vi "Load JSON Double.vi"(7 "Element":string, 8 "error in (no error)":errorcluster, 10 "Section":string, 11 "JSON string":string) -> (0 "error out":errorcluster, 3 "value":dbl)   [LabVIEW 2026, in "Settings Service.lvclass"]
uses:
  Settings Service.lvclass
  Settings Service.lvclass/Settings Service.ctl
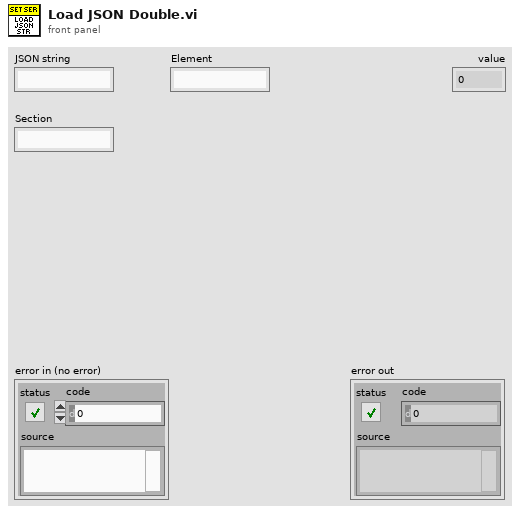
[diagram p1: front panel]
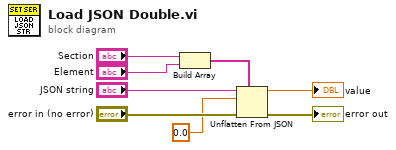
[diagram p0: block diagram]
diagram:
  n1 = Build Array("Section", "Element") -> (w4:string[])
  n2 = Unflatten From JSON(path=w4, JSON string="JSON string", type and defaults=0.0, error in (no error)="error in (no error)") -> (value=→"value":dbl, error out=→"error out":errorcluster)  [unwired: 3 in]
